vi "rasfork.vi"() -> ()   [LabVIEW 2015]
uses:
  GlobalData.vi
  GlobalPath.vi
  <vilib>/Utility/file.llb/Read Delimited Spreadsheet (string).vi
  <vilib>/Utility/file.llb/Write Delimited Spreadsheet (DBL).vi
panel:
  in  "Run Rasfork Gui":bool
  out "standard output 2":string
  out "standard output":string
  in  "c-ccd 5":bool caption="Prepare all the components (rasfork, rasfork acquisition board, calirasfork, \nbase of rasfork, weight), connect the rasfork to the board and the board to the RJ45 cable"
  in  "c-ccd 4":bool caption="Screw the 10 grey supports on each PCB side"
  in  "driver off":bool caption="Disconnect the driver from the power supply"
  out "PanelName":string
  out "appended path":path
  out "Y Diff10":dbl format="%.2f"
  out "Y Diff9":dbl format="%.2f"
  out "Y Diff8":dbl format="%.2f"
  out "Y Diff7":dbl format="%.2f"
  out "Y Diff6":dbl format="%.2f"
  out "Y Diff5":dbl format="%.2f"
  out "Y Diff4":dbl format="%.2f"
  out "Y Diff3":dbl format="%.2f"
  out "Y Diff2":dbl format="%.2f"
  out "Y Diff1":dbl format="%.2f"
  out "X Diff10":dbl format="%.2f"
  out "X Diff9":dbl
  out "X Diff8":dbl format="%.2f"
  out "X Diff7":dbl format="%.2f"
  out "X Diff6":dbl format="%.2f"
  out "X Diff5":dbl format="%.2f"
  out "X Diff4":dbl format="%.2f"
  out "X Diff3":dbl format="%.2f"
  out "X Diff2":dbl format="%.2f"
  out "X Diff1":dbl format="%.2f"
  out "all rows":string[][](array[string])
  out "Y D10":dbl format="%.2f"
  out "Y D9":dbl format="%.2f"
  out "Y D8":dbl format="%.2f"
  out "Y D7":dbl format="%.2f"
  out "Y D6":dbl format="%.2f"
  out "Y D5":dbl format="%.2f"
  out "Y D4":dbl format="%.2f"
  out "Y D3":dbl format="%.2f"
  out "Y D2":dbl format="%.2f"
  out "Y D1":dbl format="%.2f"
  out "X D10":dbl format="%.2f"
  out "X D9":dbl format="%.2f"
  out "X D8":dbl format="%.2f"
  out "X D7":dbl format="%.2f"
  out "X D6":dbl format="%.2f"
  out "X D5":dbl format="%.2f"
  out "X D4":dbl format="%.2f"
  out "X D3":dbl format="%.2f"
  out "X D2":dbl format="%.2f"
  out "X D1":dbl format="%.2f"
  out "y 6":string
  out "y 10":string
  out "y 9":string
  out "y 8":string
  out "y 7":string
  out "y 5":string
  out "y 4":string
  out "y 3":string
  out "y 2":string
  out "y 1":string
  out "x 6":string
  out "x 10":string
  out "x 9":string
  out "x 8":string
  out "x 7":string
  out "x 5":string
  out "x 4":string
  out "x 3":string
  out "x 2":string
  out "x 1":string
  out "output file":path=path "/home/atlas/Micromegas/ProdData/C_CCD/CalcDiscr.txt"
  out "Filename selected":path
  in  "Done?":bool
  out "Latest file:":path
  in  "Run Rasfork exec":bool
  in  "c-ccd 3":bool caption="Setup the electronics for the Rasfork reading:\n- make sure the ethernet cables are connected on the minimal heads\n- check that the cables connecting the driver with the muxs are plugged in\n- CONNECT the driver to the power supply and check that it is connected to the LAN"
  in  "c-ccd":bool caption="Read the data file"
  # "Rasfork reading"
  # "Type \"Table\" or \"Stiffback\" for the C-CCDs you want to use:"
  # "Run the Rasfork software"
  # "Data file reading"
  # "The most recent data file created by the C-CCD program will be opened.\nOnce the \"read data file\" is clicked, the raw data and displacement should appear on the PCB schematics on the bottom."
  # "Raw Data (mm):"
  # "Calibrated position (mm):"
  # "Difference (wrt Reference reading) (um):"
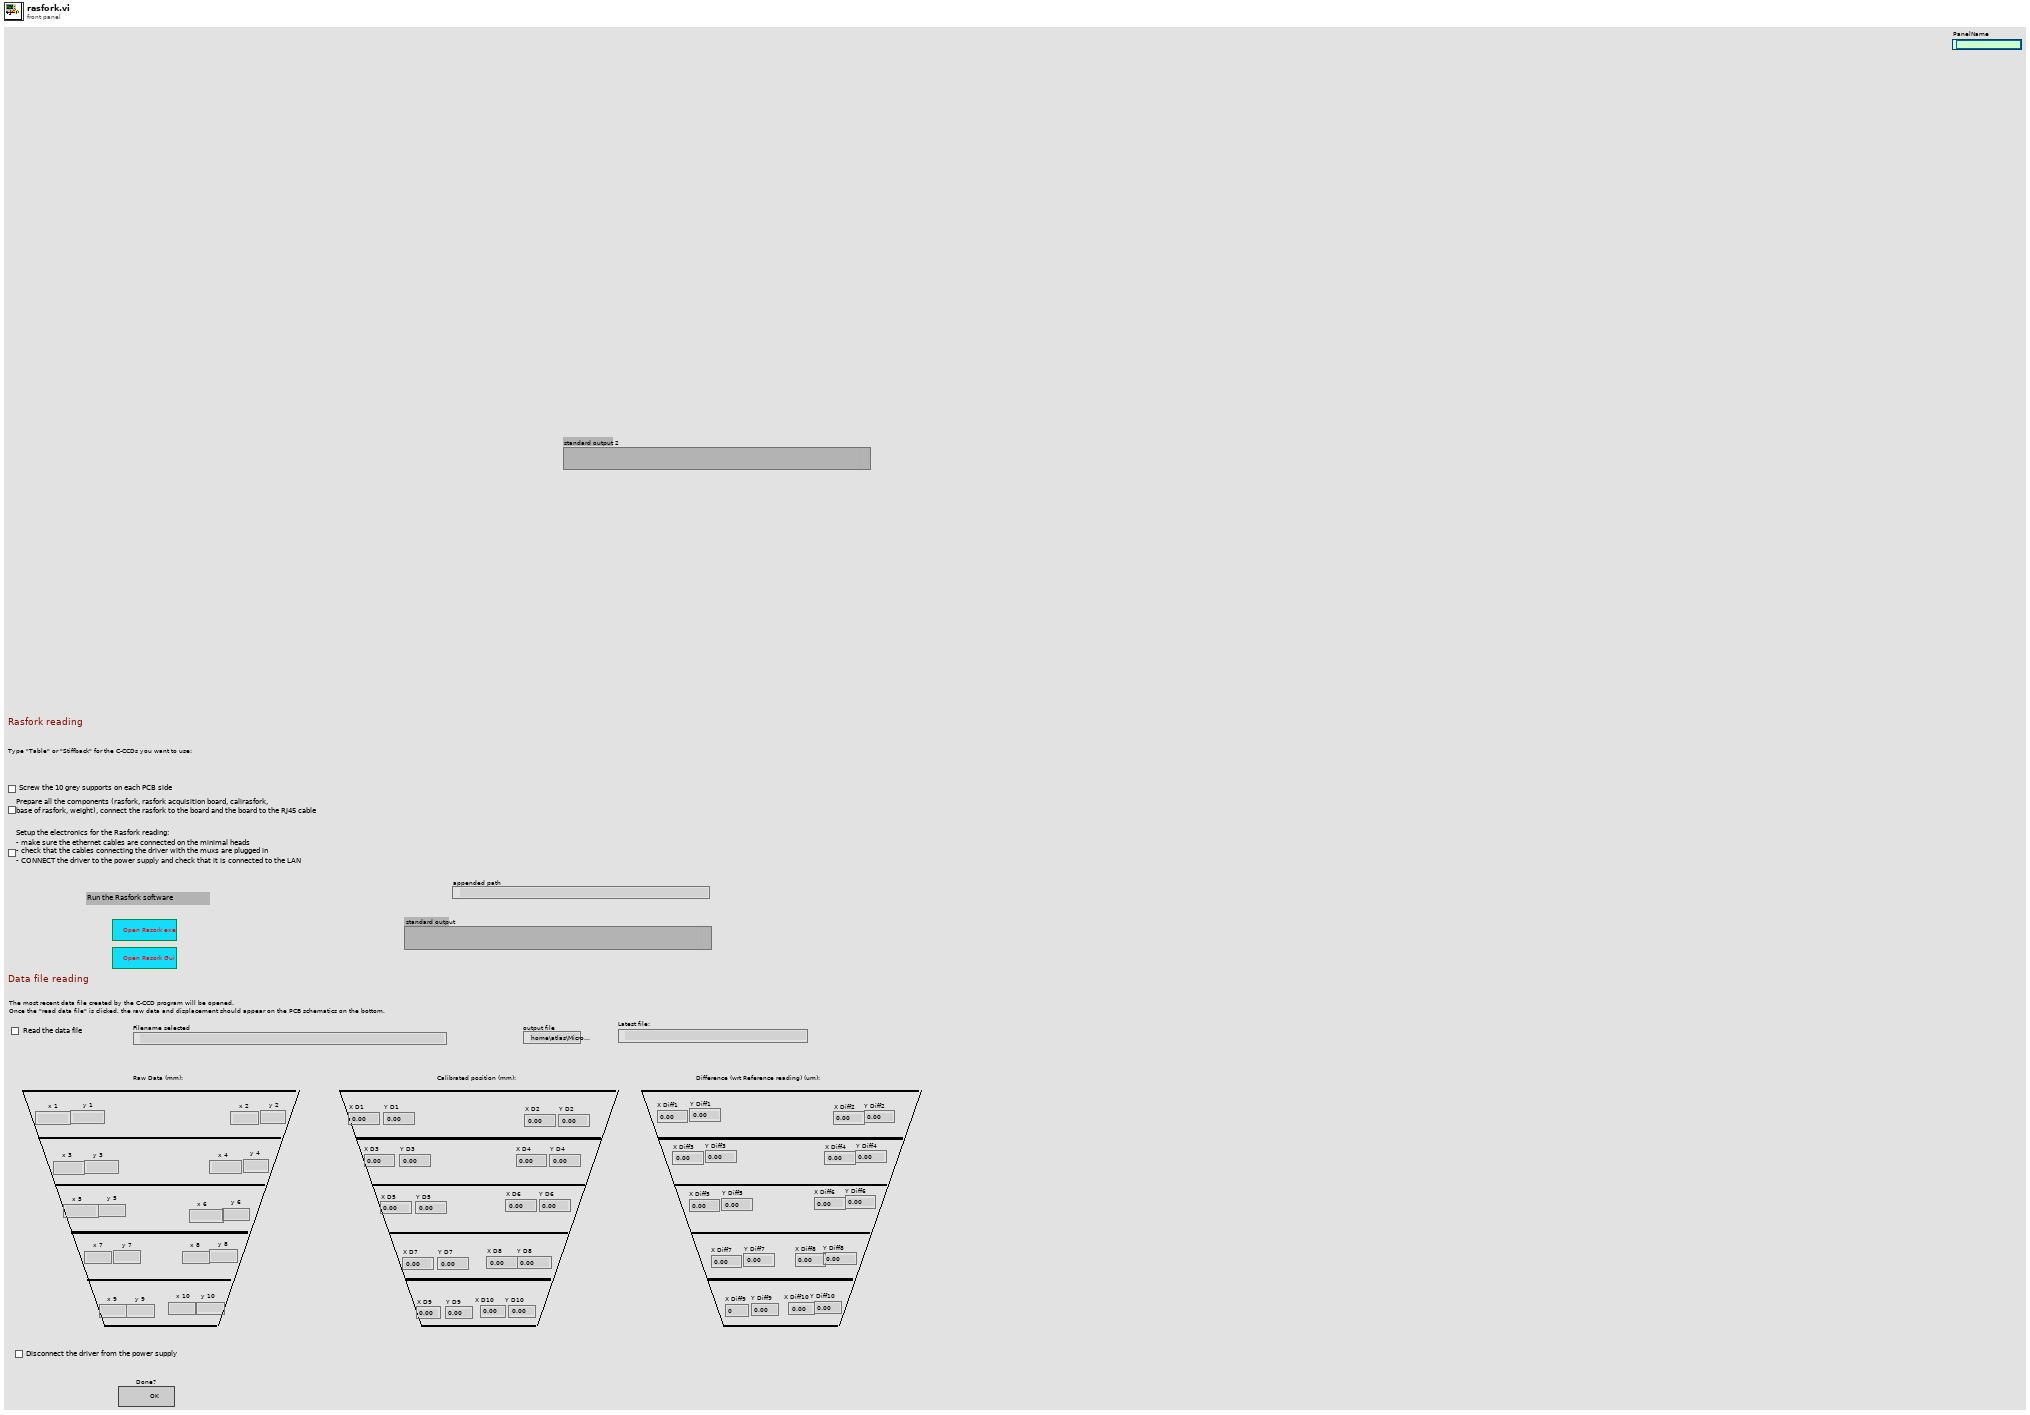
[diagram p1: front panel]
types:
  T1 = enum16{"open", "replace", "create", "open or create", "replace or create", "replace or create with confirmation"}
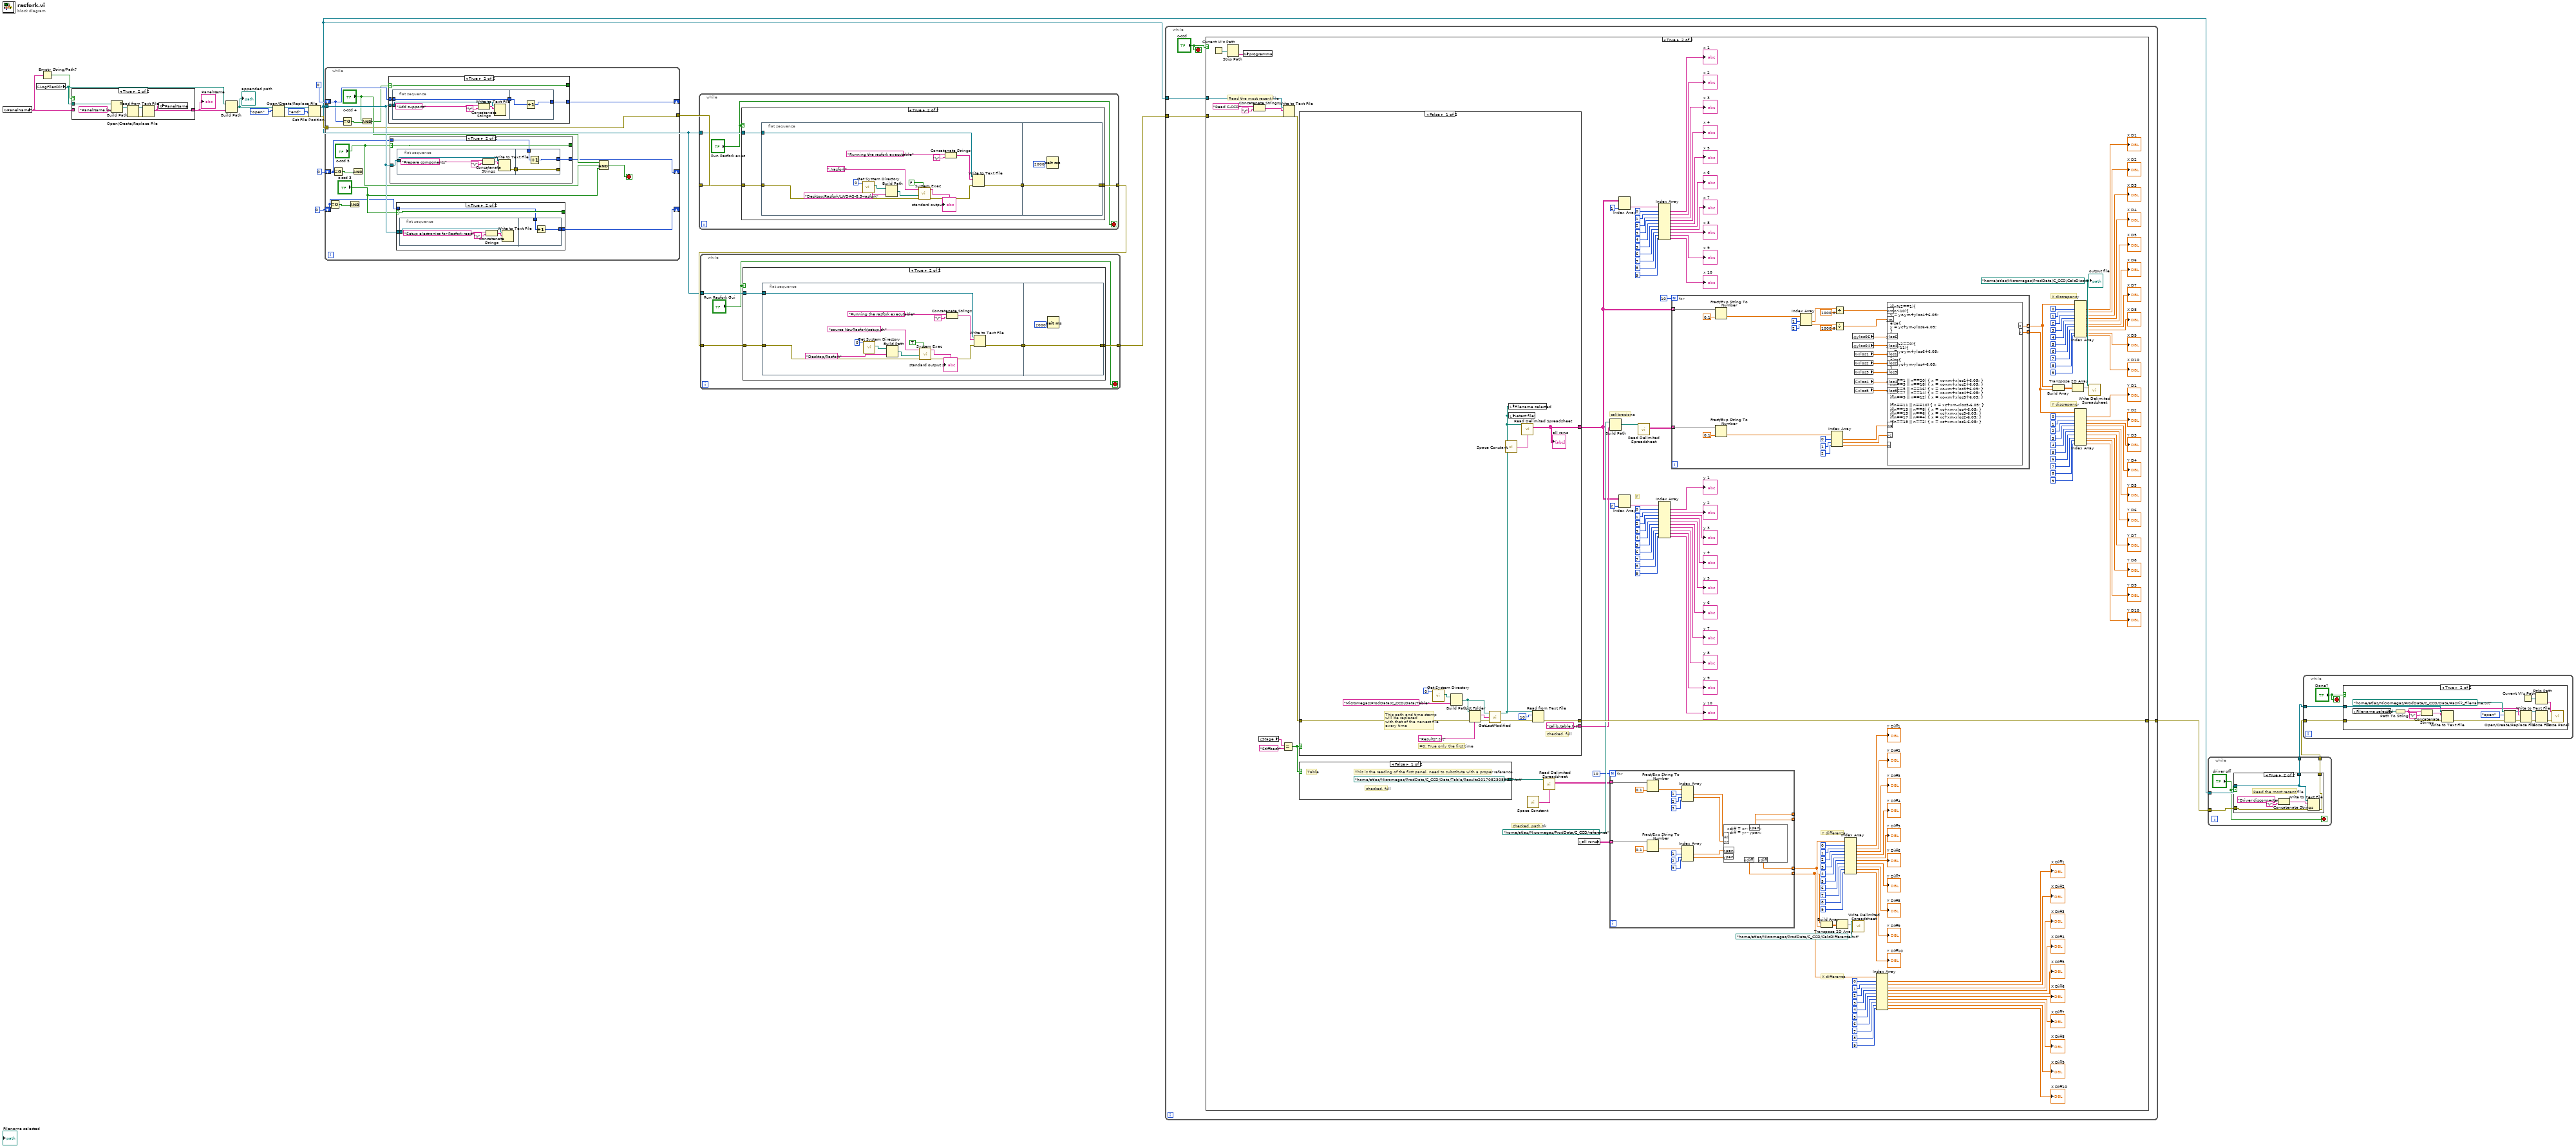
[diagram p0: block diagram]
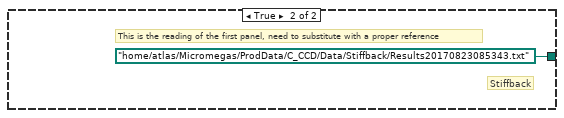
[diagram p6: hidden frame]
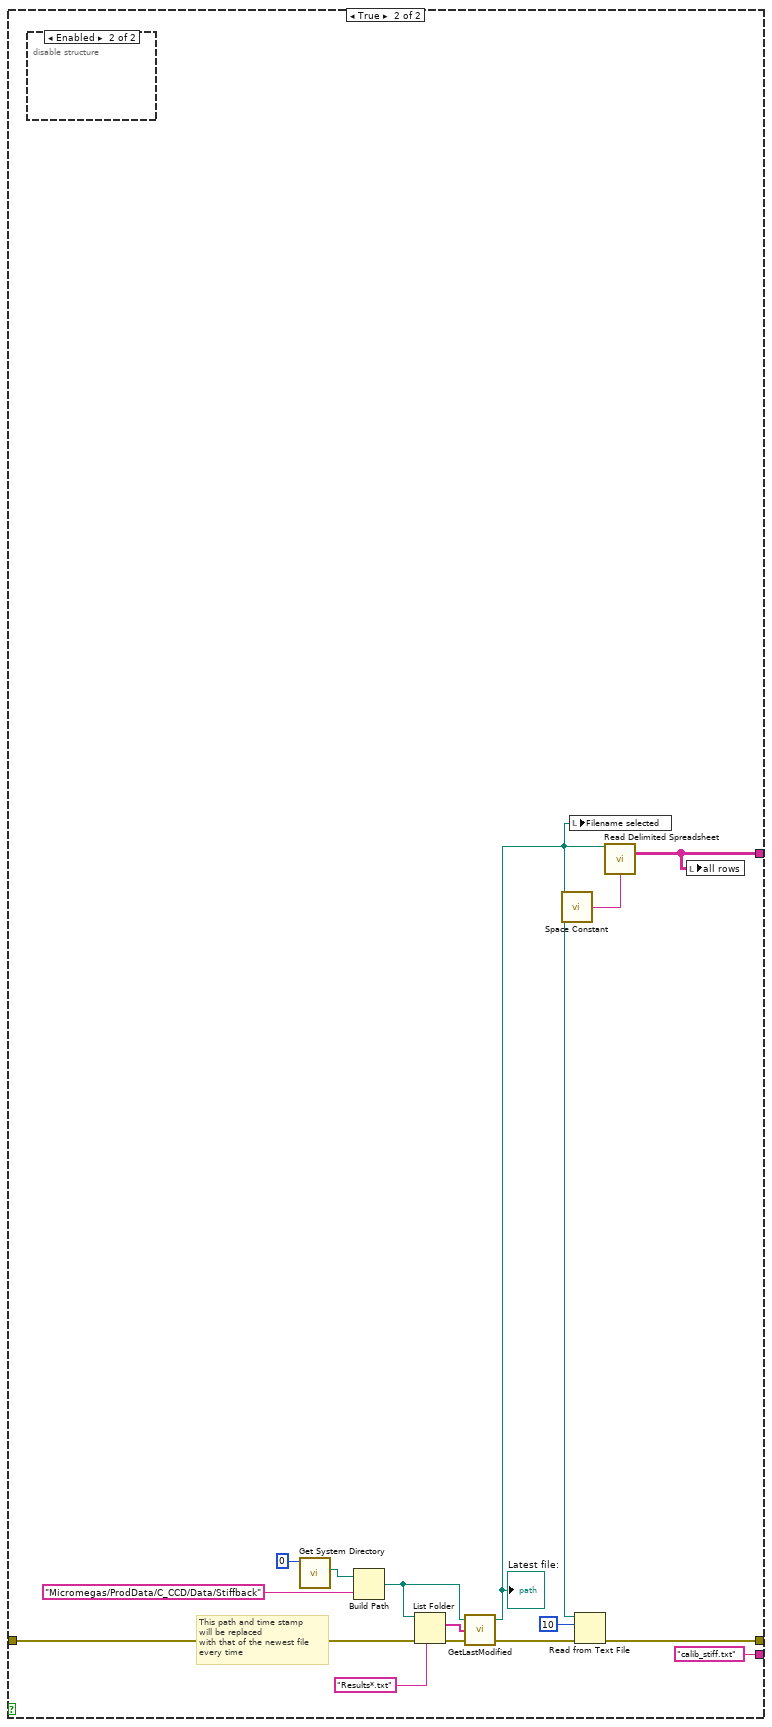
[diagram p7: hidden frame]
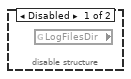
[diagram p8: hidden frame]
diagram:
  n1 = global read "GlobalData.vi" "PanelName"() -> (w17:string)
  n2 = global read "GlobalPath.vi" "LogFilesDir"() -> (w18:path)
  n3 = Empty String/Path?(string/path=w17) -> (empty?=w16:bool)
  n4 = case shown="True" w16 {
    tunnel: w18 -> [_ w27]
    tunnel: [w21 w22] -> w19
    tunnel: w17 -> [w21 _]
    frame False {
    }
    frame True {
      n5 = Build Path(base path=w27, name or relative path="PanelName.log") -> (appended path=w26:path)
      n6 = Open/Create/Replace File(file path (use dialog)=w26) -> (refnum out=w23:refnum<file>, error out=w24:errorcluster)  [unwired: 5 in, 1 out]
      n7 = Read from Text File(file (use dialog)=w23, error in=w24) -> (text=w22:string)  [unwired: 2 in, 3 out]
      n8 = global write "GlobalData.vi" "PanelName"(w22) -> ()
    }
  }
  "PanelName" <- w19
  n9 = Build Path(base path=w18, name or relative path=w19) -> (appended path=w11:path)
  "appended path" <- w11
  n10 = Open/Create/Replace File(file path (use dialog)=w11, operation (0:open)=T1."open") -> (refnum out=w14:refnum<file>, error out=w15:errorcluster)  [unwired: 4 in, 1 out]
  n11 = Set File Position(refnum=w14, from (0:start)=enum16{"start", "end", "current"}."end", error in=w15) -> (refnum out=w2:refnum<file>, error out=w4:errorcluster)  [unwired: 1 in]
  n12 = while {
    tunnel: w2 -> [w43]
    tunnel: [w28] -> w20
    shift-right: [w39] -> _
    shift-left: 0 -> [w38]
    shift-right: [w29] -> _
    shift-left: 0 -> [w31]
    shift-right: [w30] -> _
    shift-left: 0 -> [w32]
    tunnel: w4 -> [w28]
    stop <- w40 stop-if-true
    n13 = Equal To 0?(x=w31) -> (x = 0?=w33:bool)
    n14 = Equal To 0?(x=w32) -> (x = 0?=w34:bool)
    n15 = Equal To 0?(x=w38) -> (x = 0?=w37:bool)
    n16 = And(y=w33) -> ()  [unwired: 1 in, 1 out]
    n17 = And(y=w34) -> ()  [unwired: 1 in, 1 out]
    n18 = And(x="c-ccd 4", y=w37) -> (x .and. y?=w35:bool)
    n19 = case shown="True" w35 {
      selector: w35 -> [w60 w65]
      tunnel: w43 -> [_ w64]
      tunnel: [w60 w65] -> _
      tunnel: w38 -> [w59 w62]
      tunnel: [w59 w61] -> w39
      frame False {
      }
      frame True {
        n20 = flat-sequence {
          tunnel: w64 -> [w68]
          tunnel: [w66] -> w63
          tunnel: w62 -> [w66]
          tunnel: w63 -> [w72]
          tunnel: [w71] -> w61
          frame #0 {
            n21 = Concatenate Strings("Add supports", "\r") -> (w67:string)
            n22 = Write to Text File(file (use dialog)=w68, text=w67) -> ()  [unwired: 2 in, 3 out]
          }
          frame #1 {
            n23 = Increment(x=w72) -> (x+1=w71:i32)
          }
        }
      }
    }
    n24 = case shown="True" "c-ccd 5" {
      selector: "c-ccd 5" -> [w45 w50]
      tunnel: w43 -> [_ w49]
      tunnel: [w45 w50] -> _
      tunnel: w32 -> [w44 w47]
      tunnel: [w44 w46] -> w30
      frame False {
      }
      frame True {
        n25 = flat-sequence {
          tunnel: w49 -> [w52]
          tunnel: [w53] -> w48
          tunnel: [w58] -> _
          tunnel: w48 -> [w58]
          tunnel: w47 -> [w57]
          tunnel: [w56] -> w46
          frame #0 {
            n26 = Concatenate Strings("Prepare components", "\r") -> (w51:string)
            n27 = Write to Text File(file (use dialog)=w52, text=w51) -> (error out=w53:errorcluster)  [unwired: 2 in, 2 out]
          }
          frame #1 {
            n28 = Increment(x=w57) -> (x+1=w56:i32)
          }
        }
      }
    }
    n29 = case shown="True" "c-ccd 3" {
      selector: "c-ccd 3" -> [w74 w78]
      tunnel: w43 -> [_ w77]
      tunnel: [w74 w78] -> _
      tunnel: w31 -> [w73 w76]
      tunnel: [w73 w75] -> w29
      frame False {
      }
      frame True {
        n30 = flat-sequence {
          tunnel: w77 -> [w80]
          tunnel: w76 -> [w84]
          tunnel: [w83] -> w75
          frame #0 {
            n31 = Concatenate Strings("Setup electronics for Rasfork reading", "\r") -> (w79:string)
            n32 = Write to Text File(file (use dialog)=w80, text=w79) -> ()  [unwired: 2 in, 3 out]
          }
          frame #1 {
            n33 = Increment(x=w84) -> (x+1=w83:i32)
          }
        }
      }
    }
    n34 = Compound Arithmetic op=AND("c-ccd 4", "c-ccd 5", "c-ccd 3") -> (w40:bool)
  }
  n35 = while {
    tunnel: w2 -> [w86]
    tunnel: w20 -> [w88]
    tunnel: [w87] -> w3
    stop <- "Run Rasfork exec" stop-if-true
    n36 = case shown="True" "Run Rasfork exec" {
      tunnel: w88 -> [w89 w93]
      tunnel: [w89 w92] -> w87
      tunnel: w86 -> [_ w91]
      frame False {
      }
      frame True {
        n37 = flat-sequence {
          tunnel: w93 -> [w107]
          tunnel: w91 -> [w105]
          tunnel: [w106] -> w90
          tunnel: [w109] -> w92
          tunnel: w90 -> [w109]
          frame #0 {
            n38 = call <vilib>:"Get System Directory.vi"("system directory type"=0) -> ("system directory"=w98:path)  [unwired: 10 in]
            n39 = Build Path(base path=w98, name or relative path="Desktop/Rasfork/LWDAQ-8.5-rasfork") -> (appended path=w96:path)
            n40 = call <vilib>:"System Exec.vi"("wait until completion? (T)"=FALSE, "error in (no error)"=w107, "working directory"=w96, "command line"="./rasfork") -> ("error out"=w101:errorcluster, "standard output"=→"standard output":string)  [unwired: 4 in, 2 out]
            n41 = Concatenate Strings("Running the rasfork executable", "\r") -> (w104:string)
            n42 = Write to Text File(file (use dialog)=w105, text=w104, error in=w101) -> (error out=w106:errorcluster)  [unwired: 1 in, 2 out]
          }
          frame #1 {
            n43 = Wait (ms)(milliseconds to wait=2000) -> ()  [unwired: 1 out]
          }
        }
      }
    }
  }
  n44 = while {
    tunnel: w2 -> [w111]
    tunnel: w3 -> [w113]
    tunnel: [w112] -> w1
    stop <- "Run Rasfork Gui" stop-if-true
    n45 = case shown="True" "Run Rasfork Gui" {
      tunnel: w113 -> [w114 w118]
      tunnel: [w114 w117] -> w112
      tunnel: w111 -> [_ w116]
      frame False {
      }
      frame True {
        n46 = flat-sequence {
          tunnel: w118 -> [w132]
          tunnel: w116 -> [w130]
          tunnel: [w131] -> w115
          tunnel: [w134] -> w117
          tunnel: w115 -> [w134]
          frame #0 {
            n47 = call <vilib>:"Get System Directory.vi"("system directory type"=0) -> ("system directory"=w123:path)  [unwired: 10 in]
            n48 = Build Path(base path=w123, name or relative path="Desktop/Rasfork") -> (appended path=w121:path)
            n49 = call <vilib>:"System Exec.vi"("wait until completion? (T)"=TRUE, "error in (no error)"=w132, "working directory"=w121, "command line"="source NswRasfork/setup.sh") -> ("error out"=w126:errorcluster, "standard output"=→"standard output 2":string)  [unwired: 4 in, 2 out]
            n50 = Concatenate Strings("Running the rasfork executable", "\r") -> (w129:string)
            n51 = Write to Text File(file (use dialog)=w130, text=w129, error in=w126) -> (error out=w131:errorcluster)  [unwired: 1 in, 2 out]
          }
          frame #1 {
            n52 = Wait (ms)(milliseconds to wait=2000) -> ()  [unwired: 1 out]
          }
        }
      }
    }
  }
  n53 = while {
    tunnel: w2 -> [w136]
    tunnel: w1 -> [w138]
    tunnel: [w137] -> w10
    stop <- "c-ccd" stop-if-true
    n54 = case shown="True" "c-ccd" {
      tunnel: w138 -> [w139 w289]
      tunnel: [w139 w287] -> w137
      tunnel: w136 -> [_ w286]
      frame False {
      }
      frame True {
        w278 = path "/home/atlas/Micromegas/ProdData/C_CCD/CalcDiscr.txt" ("file path (dialog if empty)")
        # "checked, path ok"
        # "Y differenza"
        # "X differenza"
        # "Y discrepancy"
        # "X discrepancy"
        # "Y"
        # "calibrazione"
        # "Read the most recent file"
        n55 = Current VI's Path() -> (path=w290:path)
        n56 = Strip Path(path=w290) -> (name=w291:string)  [unwired: 1 out]
        n57 = global write "GlobalData.vi" "programma"(w291) -> ()
        n58 = Concatenate Strings("Read C-CCD", "\r") -> (w296:string)
        n59 = global read "GlobalData.vi" "Stage"() -> (w292:string)
        n60 = Equal?(x=w292, y="Stiffback") -> (x = y?=w146:bool)
        n61 = Write to Text File(file (use dialog)=w286, text=w296, error in=w289) -> (error out=w288:errorcluster)  [unwired: 1 in, 2 out]
        n62 = case shown="False" w146 {
          tunnel: w288 -> [w351 w366]
          tunnel: [w361 w376] -> w287
          tunnel: [w349 w363] -> w254
          tunnel: ["calib_table.txt" "calib_stiff.txt"] -> w283
          frame False {
            # "checked, full"
            # "=0: True only the first time"
            # "This path and time stamp\nwill be replaced\nwith that of the newest file \nevery time"
            n63 = call <vilib>:"Get System Directory.vi"("system directory type"=0) -> ("system directory"=w358:path)  [unwired: 10 in]
            n64 = Build Path(base path=w358, name or relative path="Micromegas/ProdData/C_CCD/Data/Table") -> (appended path=w353:path)
            n65 = List Folder(path=w353, pattern="Results*.txt", error in=w351) -> (filenames=w356:string[], error out=w354:errorcluster)  [unwired: 1 in, 2 out]
            n66 = call "GetLastModified.vi"("error in"=w354, "filenames"=w356, "SearchDir"=w353) -> ("error out"=w355:errorcluster, "Path"=w348:path)  [unwired: 1 out]
            n67 = call <vilib>:"Space Constant.vi"() -> ("String"=w350:string)
            n68 = local write "Filename selected"(w348) -> ()
            n69 = local write "Latest file:"(w348) -> ()
            n70 = call-poly <vilib>:"Read Delimited Spreadsheet.vi"("file path (dialog if empty)"=w348, "delimiter (\\t)"=w350) -> ("all rows"=w349:string[][])  [unwired: 8 in, 5 out]
            "all rows" <- w349
            n71 = Read from Text File(file (use dialog)=w348, count=10, error in=w355) -> (error out=w361:errorcluster)  [unwired: 1 in, 3 out]
          }
          frame True {
            # "This path and time stamp\nwill be replaced\nwith that of the newest file \nevery time"
            n72 = disable-structure shown="Enabled" {
              frame Disabled {
                n73 = global read "GlobalPath.vi" "LogFilesDir"() -> ()  [unwired: 1 out]
              }
              frame Enabled {
              }
            }
            n74 = call <vilib>:"Get System Directory.vi"("system directory type"=0) -> ("system directory"=w373:path)  [unwired: 10 in]
            n75 = Build Path(base path=w373, name or relative path="Micromegas/ProdData/C_CCD/Data/Stiffback") -> (appended path=w369:path)
            n76 = List Folder(path=w369, pattern="Results*.txt", error in=w366) -> (filenames=w368:string[], error out=w367:errorcluster)  [unwired: 1 in, 2 out]
            n77 = call "GetLastModified.vi"("error in"=w367, "filenames"=w368, "SearchDir"=w369) -> ("error out"=w370:errorcluster, "Path"=w364:path)  [unwired: 1 out]
            "Latest file:" <- w364
            n78 = call <vilib>:"Space Constant.vi"() -> ("String"=w365:string)
            n79 = local write "Filename selected"(w364) -> ()
            n80 = Read from Text File(file (use dialog)=w364, count=10, error in=w370) -> (error out=w376:errorcluster)  [unwired: 1 in, 3 out]
            n81 = call-poly <vilib>:"Read Delimited Spreadsheet.vi"("file path (dialog if empty)"=w364, "delimiter (\\t)"=w365) -> ("all rows"=w363:string[][])  [unwired: 8 in, 5 out]
            n82 = local write "all rows"(w363) -> ()
          }
        }
        n83 = case shown="False" w146 {
          tunnel: [path "/home/atlas/Micromegas/ProdData/C_CCD/Data/Table/Results20170823085217.txt" ("file path (dialog if empty)") path "/home/atlas/Micromegas/ProdData/C_CCD/Data/Stiffback/Results20170823085343.txt" ("file path (dialog if empty)")] -> w191
          frame False {
            # "checked, full"
            # "This is the reading of the first panel, need to substitute with a proper reference"
            # "Table"
          }
          frame True {
            # "Stiffback"
            # "This is the reading of the first panel, need to substitute with a proper reference"
          }
        }
        n84 = call <vilib>:"Space Constant.vi"() -> ("String"=w143:string)
        n85 = call-poly <vilib>:"Read Delimited Spreadsheet.vi"("file path (dialog if empty)"=w191, "delimiter (\\t)"=w143) -> ("all rows"=w141:string[][])  [unwired: 8 in, 5 out]
        n86 = local read "all rows"() -> (w140:string[][])
        n87 = Build Path(base path=path "/home/atlas/Micromegas/ProdData/C_CCD/reference" ("file path (dialog if empty)"), name or relative path=w283) -> (appended path=w284:path)
        n88 = for {
          N: 10 -> [_]
          tunnel: w141 -> [w316] mode=indexing
          tunnel: w140 -> [w315] mode=indexing
          tunnel: [w304] -> w168 mode=indexing
          tunnel: [w303] -> w147 mode=indexing
          tunnel: [w300] -> _ mode=indexing
          tunnel: [w299] -> _ mode=indexing
          n89 = Fract/Exp String To Number(string=w316, default (0 dbl)=0.1 ("default (0 DBL)")) -> (number=w318:dbl[])  [unwired: 2 in, 1 out]
          n90 = Fract/Exp String To Number(string=w315, default (0 dbl)=0.1 ("default (0 DBL)")) -> (number=w317:dbl[])  [unwired: 2 in, 1 out]
          n91 = Index Array(array=w318, index #1=1, index #2=2, index #3=3) -> (element #1=w308:dbl, element #2=w307:dbl)  [unwired: 1 out]
          n92 = Index Array(array=w317, index #1=1, index #2=2, index #3=3) -> (element #1=w305:dbl, element #2=w306:dbl)  [unwired: 1 out]
          n93 = formula code="xdiff = xr - xpan;\nydiff = yr - ypan;"("xr"=w308, "yr"=w307, "xpan"=w305, "ypan"=w306) -> ("xdiff"=w304:dbl, "ydiff"=w303:dbl, "xr"=w300:dbl, "xpan"=w299:dbl)
        }
        n94 = Index Array(array=w254, index (col)=1 ("disabled index (col)")) -> (element=w276:string[])  [unwired: 1 in]
        n95 = Index Array(array=w254, index (col)=2 ("disabled index (col)")) -> (element=w243:string[])  [unwired: 1 in]
        n96 = call-poly <vilib>:"Read Delimited Spreadsheet.vi"("file path (dialog if empty)"=w284) -> ("all rows"=w282:string[][])  [unwired: 9 in, 5 out]
        n97 = Index Array(array=w276, index #1=0, index #2=1, index #3=2, index #4=3, index #5=4, index #6=5, index #7=6, index #8=7, index #9=8, index #10=9) -> (element #1=→"x 1":string, element #2=→"x 2":string, element #3=→"x 3":string, element #4=→"x 4":string, element #5=→"x 5":string, element #6=→"x 6":string, element #7=→"x 7":string, element #8=→"x 8":string, element #9=→"x 9":string, element #10=→"x 10":string)
        n98 = Index Array(array=w243, index #1=0, index #2=1, index #3=2, index #4=3, index #5=4, index #6=5, index #7=6, index #8=7, index #9=8, index #10=9) -> (element #1=→"y 1":string, element #2=→"y 2":string, element #3=→"y 3":string, element #4=→"y 4":string, element #5=→"y 5":string, element #6=→"y 6":string, element #7=→"y 7":string, element #8=→"y 8":string, element #9=→"y 9":string, element #10=→"y 10":string)
        n99 = for {
          N: 10 -> [_]
          tunnel: w254 -> [w346] mode=indexing
          tunnel: [w345] -> w213 mode=indexing
          tunnel: [w344] -> w192 mode=indexing
          tunnel: w282 -> [w322] mode=indexing
          n100 = Fract/Exp String To Number(string=w346, default (0 dbl)=0.1 ("default (0 DBL)")) -> (number=w341:dbl[])  [unwired: 2 in, 1 out]
          n101 = Fract/Exp String To Number(string=w322, default (0 dbl)=0.1 ("default (0 DBL)")) -> (number=w326:dbl[])  [unwired: 2 in, 1 out]
          n102 = Index Array(array=w341, index #1=1, index #2=2) -> (element #1=w328:dbl, element #2=w332:dbl)
          n103 = Index Array(array=w326, index #1=0, index #2=1, index #3=2) -> (element #1=w321:dbl, element #2=w320:dbl, element #3=w319:dbl)
          n104 = Divide(x=w328, y=1000.0) -> (x/y=w329:dbl)
          n105 = Divide(x=w332, y=1000.0) -> (x/y=w333:dbl)
          n106 = global read "GlobalData.vi" "ylos06"() -> (w335:dbl)
          n107 = global read "GlobalData.vi" "ylos04"() -> (w334:dbl)
          n108 = global read "GlobalData.vi" "xlos1"() -> (w340:dbl)
          n109 = global read "GlobalData.vi" "xlos2"() -> (w339:dbl)
          n110 = global read "GlobalData.vi" "xlos3"() -> (w338:dbl)
          n111 = global read "GlobalData.vi" "xlos4"() -> (w337:dbl)
          n112 = global read "GlobalData.vi" "xlos5"() -> (w336:dbl)
          n113 = formula code="if(n%2==1){\nif(n<10){\ny = yc-ym+ylos4+6.05;\n}\nelse{\ny = yc+ym-ylos6-6.05;\n}\n}\n\nif(n%2==0){\nif(n<11){\ny = yc-ym+ylos6+6.05;\n}\nelse{\ny = yc+ym-ylos4-6.05;\n}\n}\n\nif(n==1 || n==20) { x = xc-xm+xlos1+6.05; } \nif(n==3 || n==18) { x = xc-xm+xlos2+6.05; }\nif(n==5 || n==16) { x = xc-xm+xlos3+6.05; }\nif(n==7 || n==14) { x = xc-xm+xlos4+6.05; }\nif(n==9 || n==12) { x = xc-xm+xlos5+6.05; }\n\nif(n==11 || n==10) { x = xc+xm-xlos5-6.05; } \nif(n==13 || n==8) { x = xc+xm-xlos4-6.05; }\nif(n==15 || n==6) { x = xc+xm-xlos3-6.05; }\nif(n==17 || n==4) { x = xc+xm-xlos2-6.05; }\nif(n==19 || n==2) { x = xc+xm-xlos1-6.05; }"("xm"=w329, "ym"=w333, "ylos6"=w335, "ylos4"=w334, "xlos1"=w340, "xlos2"=w339, "xlos3"=w338, "xlos4"=w337, "xlos5"=w336, "xc"=w321, "yc"=w320, "n"=w319) -> ("x"=w345:dbl, "y"=w344:dbl)
        }
        n114 = Build Array(w168, w147) -> (w144:dbl[][])
        n115 = Transpose 2D Array(2D array=w144) -> (transposed array=w142:dbl[][])
        n116 = Index Array(array=w147, index #1=0, index #2=1, index #3=2, index #4=3, index #5=4, index #6=5, index #7=6, index #8=7, index #9=8, index #10=9) -> (element #1=→"Y Diff1":dbl, element #2=→"Y Diff2":dbl, element #3=→"Y Diff3":dbl, element #4=→"Y Diff4":dbl, element #5=→"Y Diff5":dbl, element #6=→"Y Diff6":dbl, element #7=→"Y Diff7":dbl, element #8=→"Y Diff8":dbl, element #9=→"Y Diff9":dbl, element #10=→"Y Diff10":dbl)
        n117 = call-poly <vilib>:"Write Delimited Spreadsheet.vi"("file path (dialog if empty)"=path "/home/atlas/Micromegas/ProdData/C_CCD/CalcDifferenza.txt", "2D data"=w142) -> ()  [unwired: 12 in, 2 out]
        n118 = Index Array(array=w168, index #1=0, index #2=1, index #3=2, index #4=3, index #5=4, index #6=5, index #7=6, index #8=7, index #9=8, index #10=9) -> (element #1=→"X Diff1":dbl, element #2=→"X Diff2":dbl, element #3=→"X Diff3":dbl, element #4=→"X Diff4":dbl, element #5=→"X Diff5":dbl, element #6=→"X Diff6":dbl, element #7=→"X Diff7":dbl, element #8=→"X Diff8":dbl, element #9=→"X Diff9":dbl, element #10=→"X Diff10":dbl)
        n119 = Build Array(w213, w192) -> (w280:dbl[][])
        n120 = Transpose 2D Array(2D array=w280) -> (transposed array=w279:dbl[][])
        n121 = Index Array(array=w213, index #1=0, index #2=1, index #3=2, index #4=3, index #5=4, index #6=5, index #7=6, index #8=7, index #9=8, index #10=9) -> (element #1=→"X D1":dbl, element #2=→"X D2":dbl, element #3=→"X D3":dbl, element #4=→"X D4":dbl, element #5=→"X D5":dbl, element #6=→"X D6":dbl, element #7=→"X D7":dbl, element #8=→"X D8":dbl, element #9=→"X D9":dbl, element #10=→"X D10":dbl)
        n122 = Index Array(array=w192, index #1=0, index #2=1, index #3=2, index #4=3, index #5=4, index #6=5, index #7=6, index #8=7, index #9=8, index #10=9) -> (element #1=→"Y D1":dbl, element #2=→"Y D2":dbl, element #3=→"Y D3":dbl, element #4=→"Y D4":dbl, element #5=→"Y D5":dbl, element #6=→"Y D6":dbl, element #7=→"Y D7":dbl, element #8=→"Y D8":dbl, element #9=→"Y D9":dbl, element #10=→"Y D10":dbl)
        n123 = call-poly <vilib>:"Write Delimited Spreadsheet.vi"("file path (dialog if empty)"=w278, "2D data"=w279) -> ()  [unwired: 12 in, 2 out]
        "output file" <- w278
      }
    }
  }
  n124 = while {
    tunnel: w2 -> [w382]
    tunnel: w10 -> [w381]
    tunnel: [w380] -> w9
    tunnel: [w379] -> w8
    stop <- "driver off" stop-if-true
    n125 = case shown="True" "driver off" {
      tunnel: w382 -> [w384 w386]
      tunnel: w381 -> [w383 w387]
      tunnel: [w384 w386] -> w380
      tunnel: [w383 w385] -> w379
      frame False {
      }
      frame True {
        # "Read the most recent file"
        n126 = Concatenate Strings("Driver disconnected", "\r") -> (w390:string)
        n127 = Write to Text File(file (use dialog)=w386, text=w390, error in=w387) -> (error out=w385:errorcluster)  [unwired: 1 in, 2 out]
      }
    }
  }
  n128 = while {
    tunnel: w8 -> [w392]
    tunnel: w9 -> [w391]
    stop <- "Done?" stop-if-true
    n129 = case shown="True" "Done?" {
      tunnel: w392 -> [_ w397]
      tunnel: w391 -> [_ w396]
      frame False {
      }
      frame True {
        n130 = local read "Filename selected"() -> (w398:path)
        n131 = Path To String(path=w398) -> (string=w404:string)
        n132 = Concatenate Strings(w404, "\r") -> (w405:string)
        n133 = Write to Text File(file (use dialog)=w396, text=w405, error in=w397) -> (error out=w394:errorcluster)  [unwired: 1 in, 2 out]
        n134 = Open/Create/Replace File(file path (use dialog)=path "/home/atlas/Micromegas/ProdData/C_CCD/Data/Rasnik_Filename.txt", error in=w394, operation (0:open)=T1."open") -> (refnum out=w403:refnum<file>, error out=w400:errorcluster)  [unwired: 3 in, 1 out]
        n135 = Write to Text File(file (use dialog)=w403, text=w404, error in=w400) -> (refnum out=w402:refnum<file>, error out=w401:errorcluster)  [unwired: 1 in, 1 out]
        n136 = Current VI's Path() -> (path=w408:path)
        n137 = Strip Path(path=w408) -> (name=w409:string)  [unwired: 1 out]
        n138 = Close File(refnum=w402, error in=w401) -> (error out=w395:errorcluster)  [unwired: 1 out]
        n139 = call <vilib>:"Close Panel.vi"("error in (no error)"=w395, "VI name"=w409) -> ()  [unwired: 9 in, 1 out]
      }
    }
  }
